vi "DTMF.vi"() -> ()   [LabVIEW 2020]
uses:
  <vilib>/Waveform/WDTOps.llb/WDT Index Channel DBL.vi
  <vilib>/express/express analysis/Spectral/Block/exnSpectralBlock spectral measurements RMS poly.vi
  <vilib>/express/express analysis/Spectral/Block/exnSpectralBlock spectral measurements RMS array WFM.vi
  <vilib>/express/express analysis/Spectral/XNode/ExpressSpectralMeasurementsBlockNode.xnode
  <vilib>/Analysis/NI_AAL_SigProc.lvlib
  <vilib>/Analysis/NI_AALPro.lvlib
panel:
  out "digitzed pulses":waveform(dbl)(graph)
  out "DTMF Number":string
  out "derivative of digitized pulses to determine DTMF tone locations":dbl[](graph)
  out "cleaner DC pulse, applied low pass with 40Hz cut off":dynamicdata(graph)
  out "filtered abs waveform graph":waveform(dbl)[](graph)
  out "Power Spectrum filtered":dynamicdata(graph)
  out "filtered Waveform Graph":waveform(dbl)[](graph)
  out "Power Spectrum of single digit (last)":cluster{"f0":dbl, "df":dbl, "magnitude":dbl[]}[](graph)
  out "Raw Waveform Graph":waveform(dbl)[](graph)
  in  "Wav Path":path
  # "This program is for Offline decoding of a series DTMF tone"
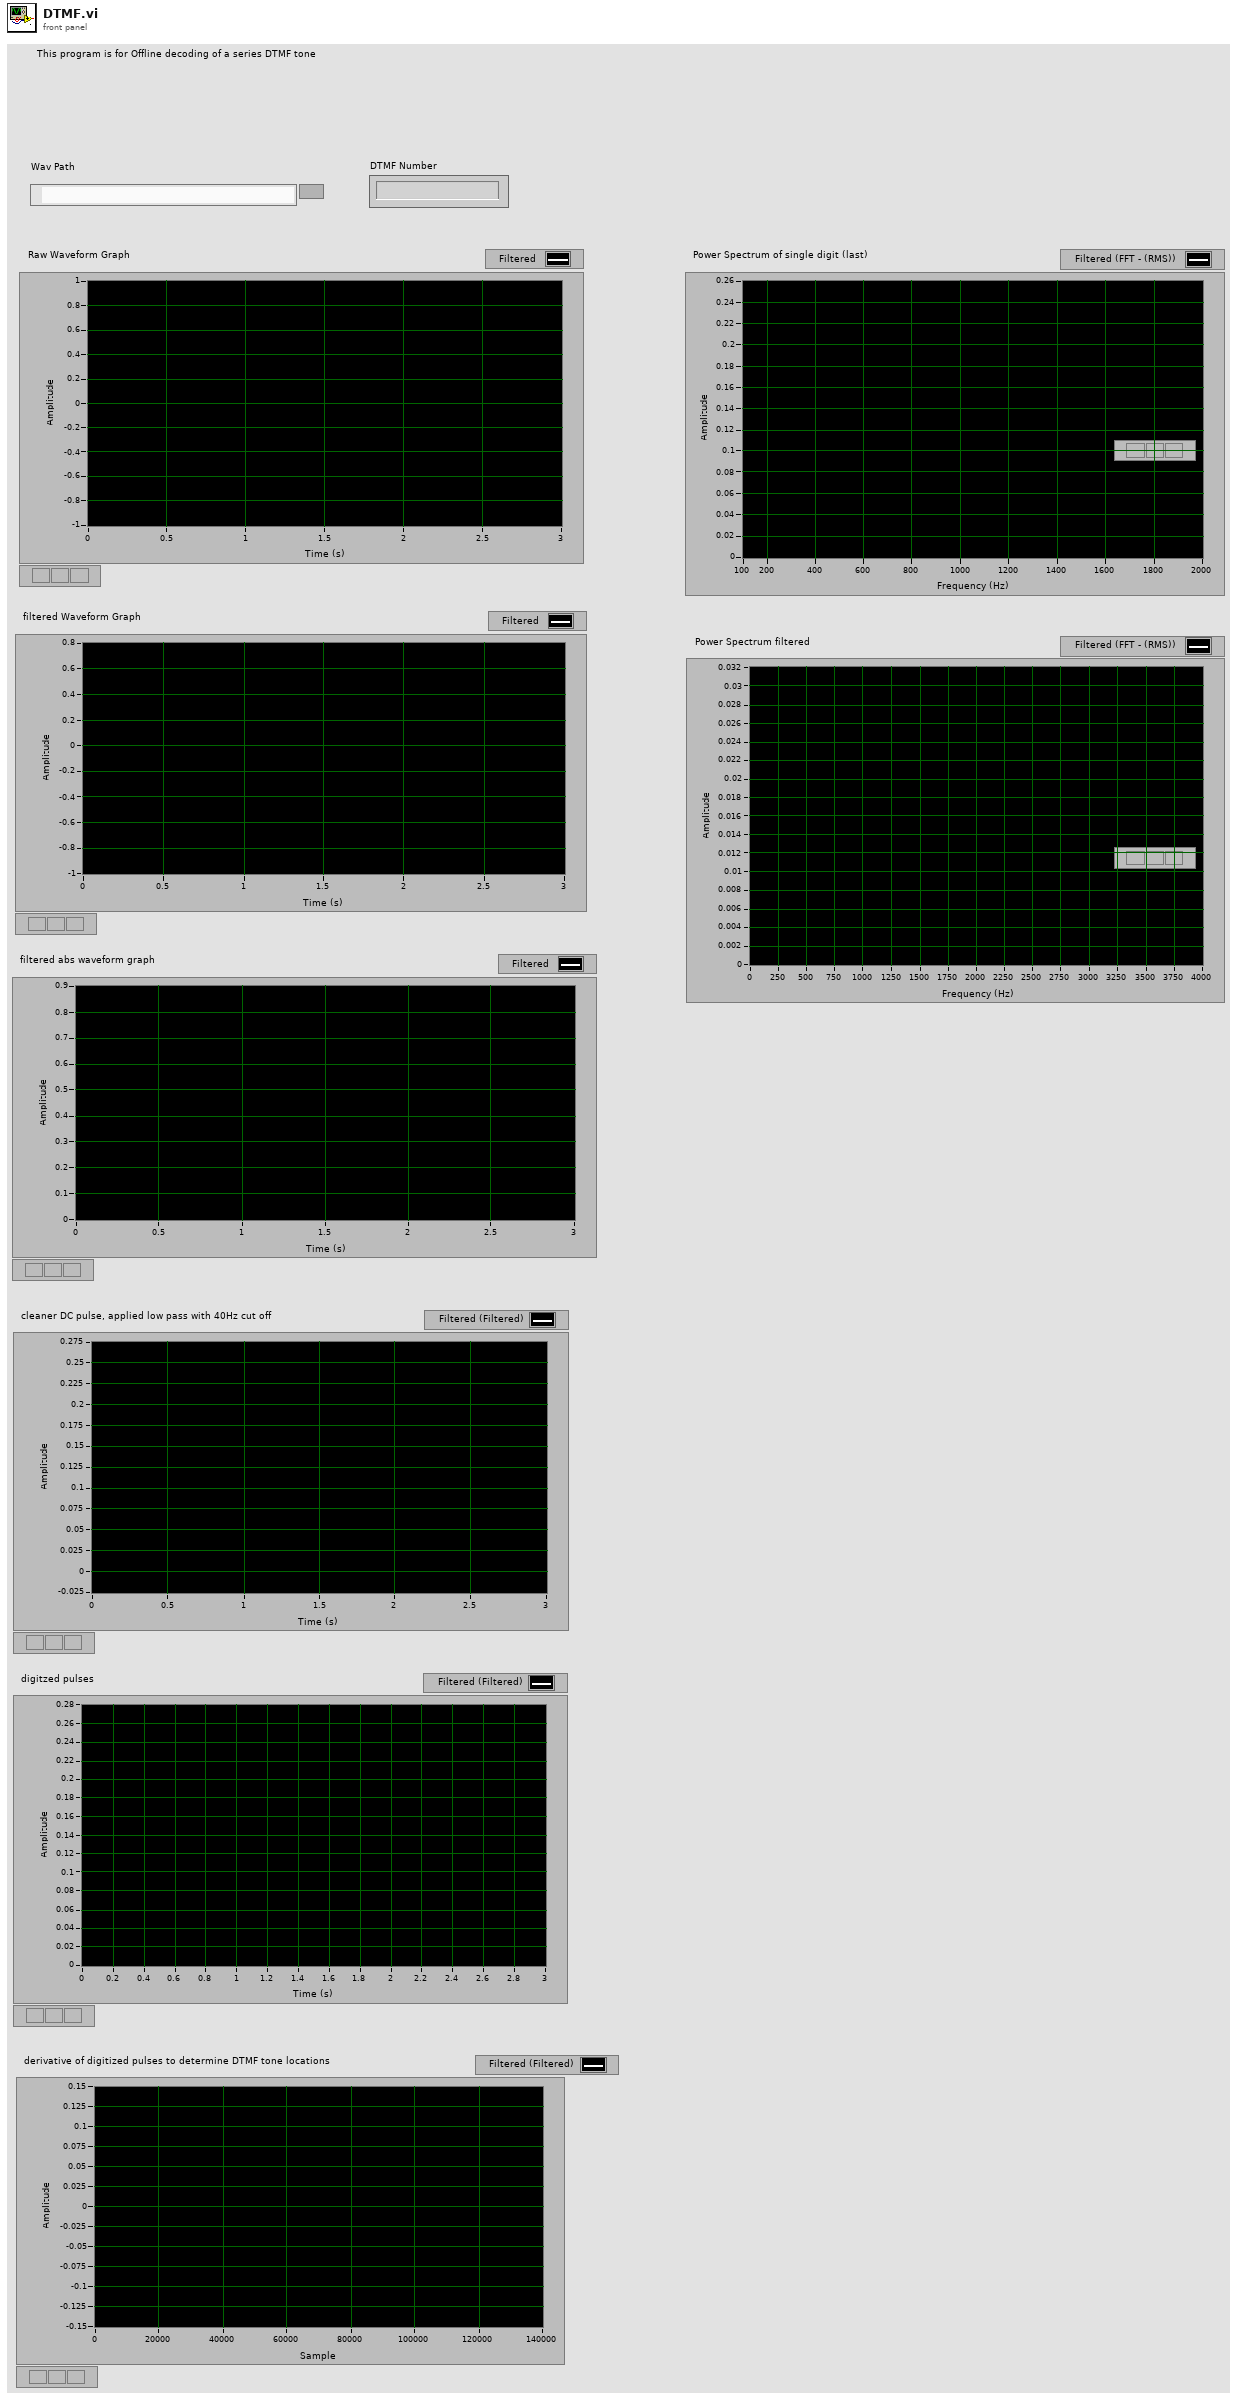
[diagram p1: front panel]
types:
  T1 = cluster{"averaging mode":u16, "weighting mode":u16, "number of averages":u32}
  T2 = cluster{"dB On (F)":bool, "unwrap phase (F)":bool, "convert to degree (F)":bool}
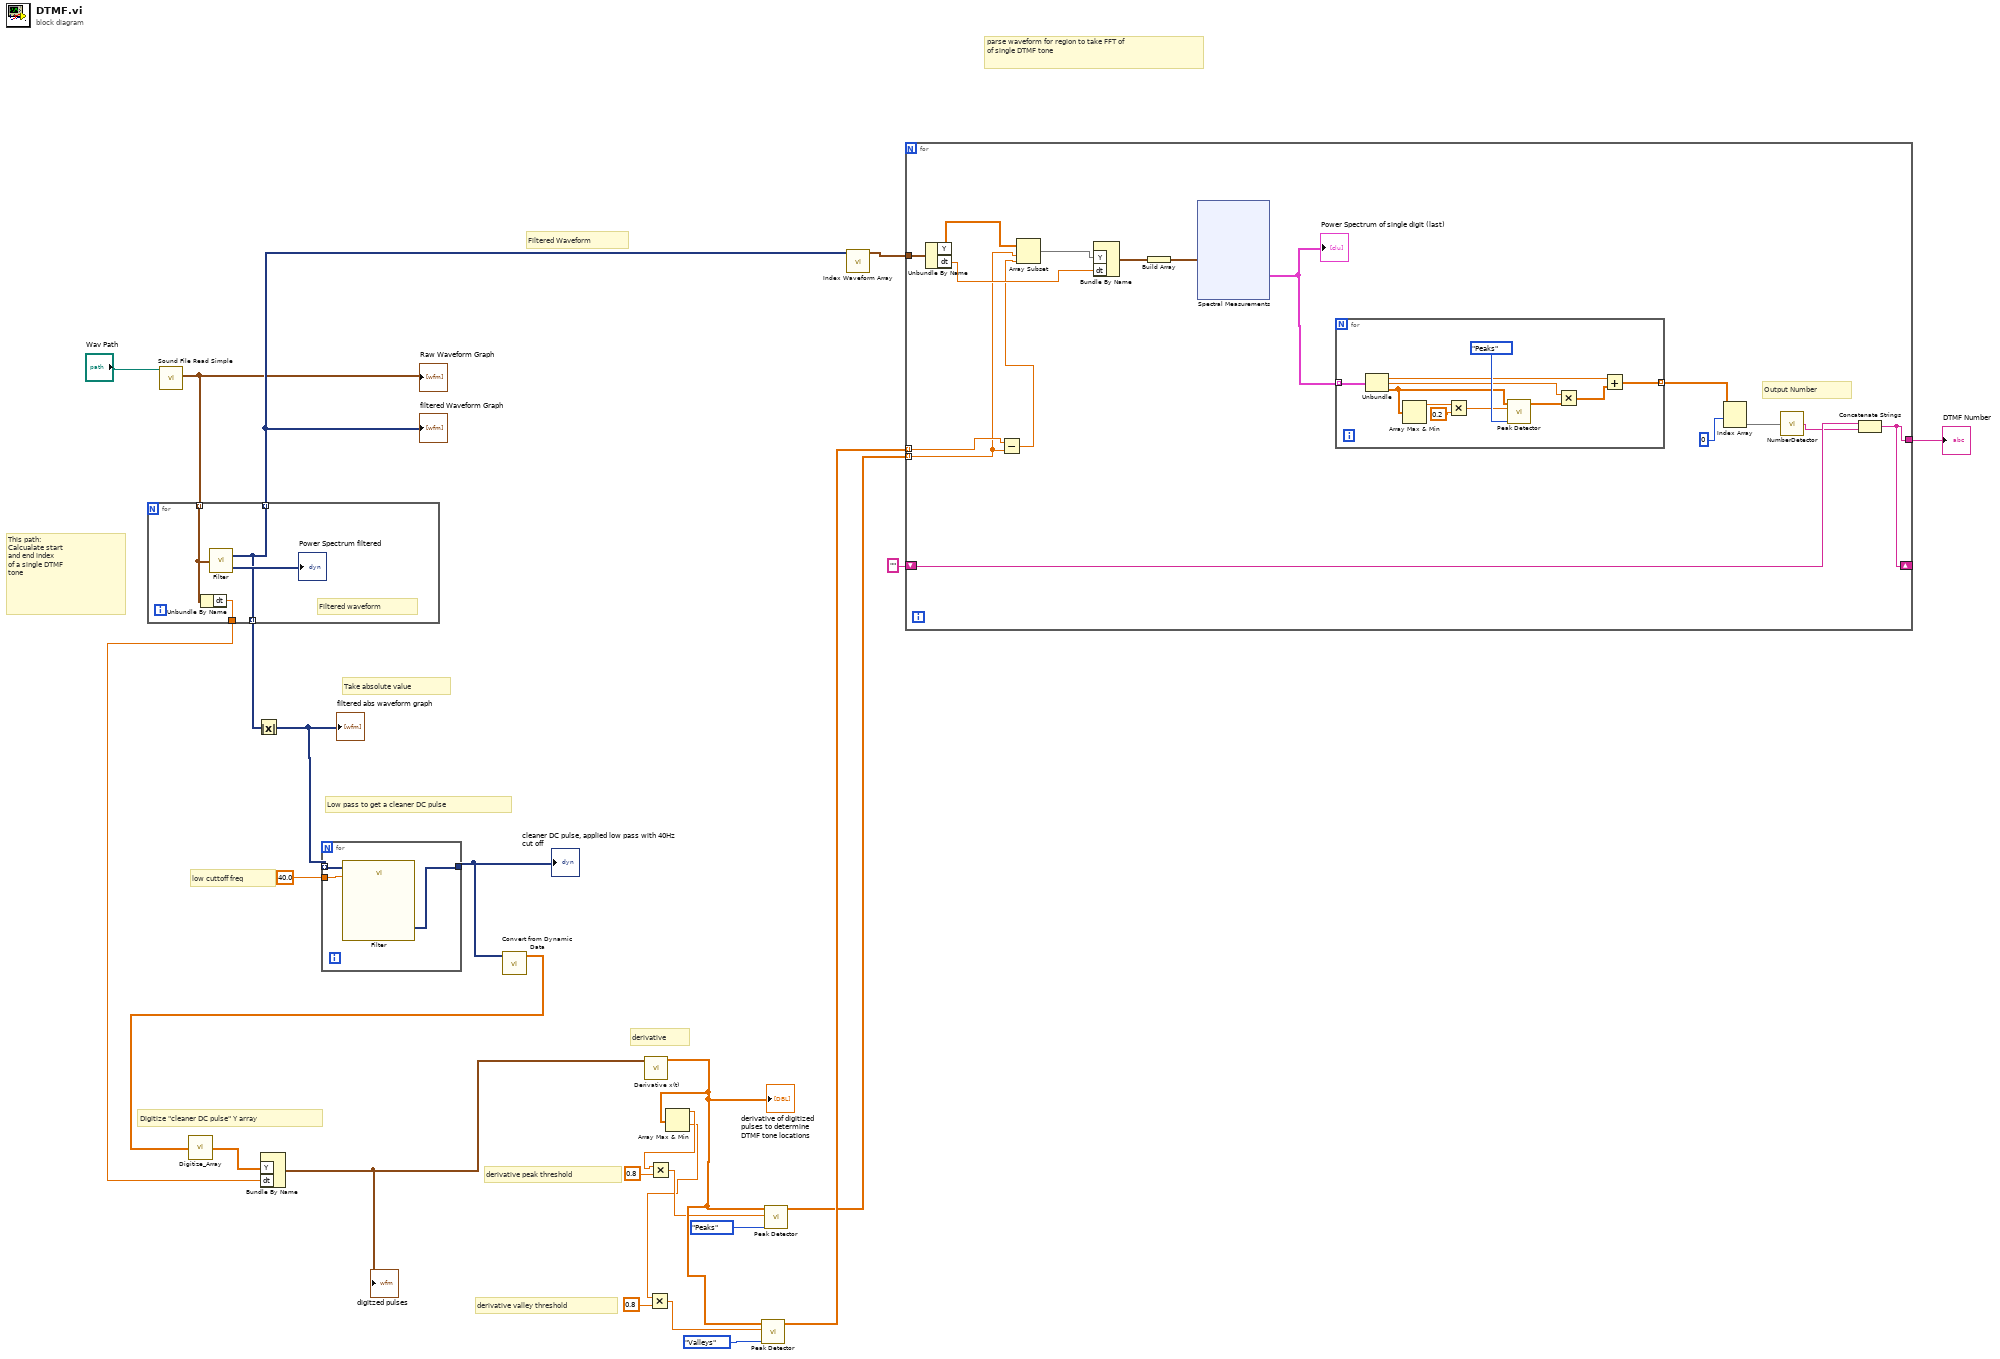
[diagram p0: block diagram]
diagram:
  # "low cuttoff freq"
  # "Filtered Waveform"
  # "Digitize \"cleaner DC pulse\" Y array"
  # "parse waveform for region to take FFT of\nof single DTMF tone"
  # "derivative valley threshold"
  # "derivative peak threshold"
  # "derivative"
  # "This path: \nCalcualate start\nand end index\nof a single DTMF\ntone"
  # "Low pass to get a cleaner DC pulse"
  # "Take absolute value"
  n1 = call <vilib>:"Sound File Read Simple.vi"("path"="Wav Path") -> ("data"=w9:waveform(dbl)[])  [unwired: 7 in, 3 out]
  "Raw Waveform Graph" <- w9
  n2 = for {
    tunnel: w9 -> [w27] mode=indexing
    tunnel: [w28] -> w22 mode=indexing
    tunnel: [w28] -> w24 mode=indexing
    tunnel: [w26] -> w7
    # "Filtered waveform"
    n3 = Unbundle By Name(w27) -> ("dt"=w26:dbl)
    n4 = call "Filter.vi"("data"=w27) -> ("Dynamic Data"=w28:dynamicdata, "FFT - (RMS)"=→"Power Spectrum filtered":dynamicdata)
  }
  "filtered Waveform Graph" <- w22
  n5 = Absolute Value(x=w24) -> (abs(x)=w23:dynamicdata[])
  "filtered abs waveform graph" <- w23
  n6 = for {
    tunnel: w23 -> [w32] mode=indexing
    tunnel: [w30] -> w8
    tunnel: 40.0 ("Lower Cut-Off (Hz)") -> [w31]
    n7 = call "Filter"("Lower Cut-Off"=w31, "Signal"=w32) -> ("Filtered Signal"=w30:dynamicdata)  [unwired: 8 in, 1 out]
  }
  "cleaner DC pulse, applied low pass with 40Hz cut off" <- w8
  n8 = call "Convert from Dynamic Data"("Dynamic Data Type"=w8) -> ("Array"=w1:dbl[])  [unwired: 3 in]
  n9 = call "Digitize_Array.vi"("Array in"=w1) -> ("Array out"=w6:dbl[])
  n10 = Bundle By Name("Y"=w6, "dt"=w7) -> (w5:waveform(dbl))  [unwired: 1 in]
  "digitzed pulses" <- w5
  n11 = call <vilib>:"Derivative x(t).vi"("X"=w5) -> ("dX/dt"=w16:dbl[])  [unwired: 9 in, 1 out]
  "derivative of digitized pulses to determine DTMF tone locations" <- w16
  n12 = Array Max & Min(array=w16) -> (max value=w15:dbl, min value=w11:dbl)  [unwired: 2 out]
  n13 = Multiply(x=w11, y=0.8) -> (x*y=w10:dbl)
  n14 = Multiply(x=w15, y=0.8) -> (x*y=w13:dbl)
  n15 = call <vilib>:"Peak Detector.vi"("peaks/valleys"=enum32{"Peaks", "Valleys"}."Valleys", "threshold"=w10, "X"=w16) -> ("Locations"=w3:dbl[])  [unwired: 4 in, 4 out]
  n16 = call <vilib>:"Peak Detector.vi"("peaks/valleys"=enum32{"Peaks", "Valleys"}."Peaks", "threshold"=w13, "X"=w16) -> ("Locations"=w2:dbl[])  [unwired: 4 in, 4 out]
  n17 = call-poly <vilib>:"Index Waveform Array.vi"("waveform array"=w22) -> ("waveform"=w19:waveform(dbl))  [unwired: 9 in, 1 out]
  n18 = for {
    tunnel: w19 -> [w48]
    tunnel: w2 -> [w37] mode=indexing
    tunnel: w3 -> [w38] mode=indexing
    shift-right: [w33] -> _
    shift-left: "" -> [w35]
    tunnel: [w33] -> w18
    # "Output Number"
    n19 = Unbundle By Name(w48) -> ("Y"=w45:dbl[], "dt"=w44:dbl)
    n20 = Subtract(x=w38, y=w37) -> (x-y=w36:dbl)
    n21 = Array Subset(array=w45, index=w37, length=w36) -> (w43:dbl[])
    n22 = Bundle By Name("Y"=w43, "dt"=w44) -> (w47:waveform(dbl))  [unwired: 1 in]
    n23 = Build Array(w47) -> (w46:waveform(dbl)[])
    n24 = xnode "Spectral Measurements"("Signals"=w46) -> ("FFT - (RMS)"=w42:cluster{"f0":dbl, "df":dbl, "magnitude":dbl[]}[])  [unwired: 1 in, 2 out]
    "Power Spectrum of single digit (last)" <- w42
    n25 = for {
      tunnel: w42 -> [w59] mode=indexing
      tunnel: [w53] -> w41 mode=indexing
      n26 = Unbundle(w59) -> ("f0"=w56:dbl, "df"=w54:dbl, "magnitude"=w52:dbl[])
      n27 = Array Max & Min(array=w52) -> (max value=w51:dbl)  [unwired: 3 out]
      n28 = Multiply(x=w51, y=0.2) -> (x*y=w49:dbl)
      n29 = call <vilib>:"Peak Detector.vi"("peaks/valleys"=enum32{"Peaks", "Valleys"}."Peaks", "threshold"=w49, "X"=w52) -> ("Locations"=w55:dbl[])  [unwired: 4 in, 4 out]
      n30 = Multiply(x=w54, y=w55) -> (x*y=w57:dbl[])
      n31 = Add(x=w56, y=w57) -> (x+y=w53:dbl[])
    }
    n32 = Index Array(array=w41, index (row)=0 ("disabled index (row)")) -> (element=w39:dbl[])  [unwired: 1 in]
    n33 = call "NumberDetector.vi"("Array"=w39) -> ("f"=w34:string)
    n34 = Concatenate Strings(w35, w34) -> (w33:string)
  }
  "DTMF Number" <- w18
